vi "Write Path Data.vi"(8 "error in (no error)":errorcluster, 10 "Path.lvclass":refnum<class "Path.lvclass">, 11 "Tool Path in":refnum<class "Tool Path.lvclass">) -> (0 "error out":errorcluster, 3 "Tool Path out":refnum<class "Tool Path.lvclass">)   [LabVIEW 2019, in "Tool Path.lvclass"]
uses:
  Tool Path.lvclass
  Parse/ParsePaths/Path.lvclass
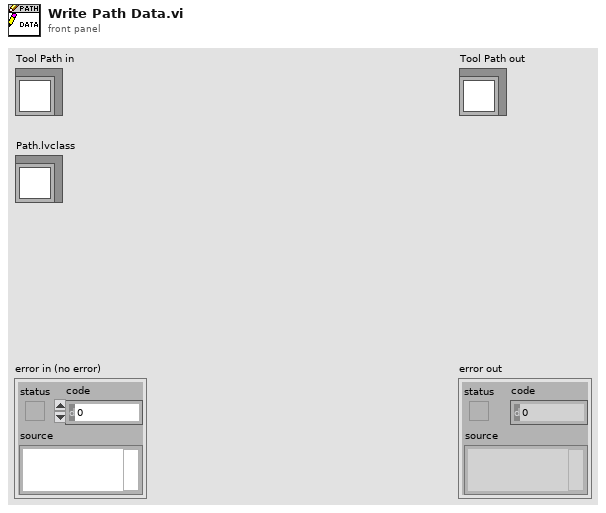
[diagram p1: front panel]
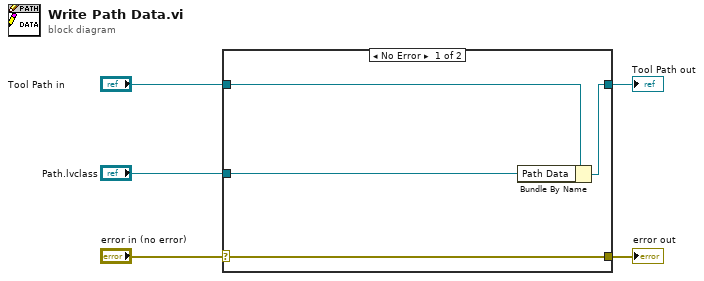
[diagram p0: block diagram]
diagram:
  n1 = case shown="No Error" "error in (no error)" {
    selector: "error in (no error)" -> [w9 w10]
    tunnel: [w9 w10] -> w4
    tunnel: [w7 w11] -> w2
    tunnel: "Tool Path in" -> [w8 w11]
    tunnel: "Path.lvclass" -> [w6 _]
    frame No Error {
      n2 = Bundle By Name(cluster=w8, "Path Data"=w6) -> (w7:refnum<class "Tool Path.lvclass">)
    }
    frame Error {
    }
  }
  "error out" <- w4
  "Tool Path out" <- w2
